vi "Between 2 Limits.vi"(8 "Lower Limit":bool, 10 "Input":dbl, 11 "Upper Limit":bool) -> (3 "Output":dbl)   [LabVIEW 2014]
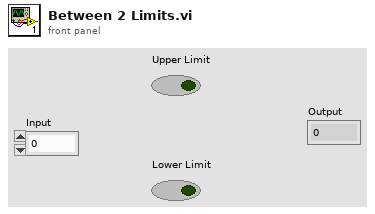
[diagram p1: front panel]
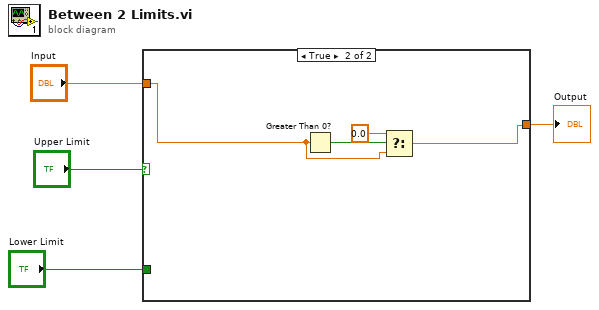
[diagram p0: block diagram]
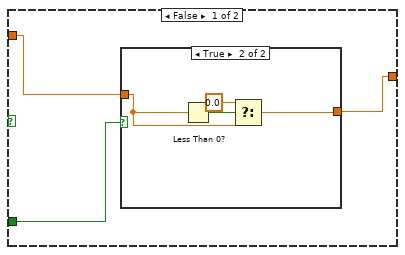
[diagram p2: hidden frame]
diagram:
  n1 = case shown="True" "Upper Limit" {
    tunnel: [w5 w15] -> w3
    tunnel: "Input" -> [w6 w14]
    tunnel: "Lower Limit" -> [w7 _]
    frame False {
      n2 = case shown="True" w7 {
        tunnel: w6 -> [w8 w9]
        tunnel: [w8 w11] -> w5
        frame False {
        }
        frame True {
          n3 = Less Than 0?(x=w9) -> (x < 0?=w12:bool)
          n4 = Select(t=0.0, s=w12, f=w9) -> (s? t:f=w11:dbl)
        }
      }
    }
    frame True {
      n5 = Greater Than 0?(x=w14) -> (x > 0?=w16:bool)
      n6 = Select(t=0.0, s=w16, f=w14) -> (s? t:f=w15:dbl)
    }
  }
  "Output" <- w3
